vi "PC_Record.vi"() -> ()   [LabVIEW 2018]
uses:
  <vilib>/Utility/inputDevices.llb/joystickAcquire.vi
  <vilib>/Utility/file.llb/Write Delimited Spreadsheet (DBL).vi
  <vilib>/Utility/inputDevices.llb/closeJoystick.vi
  <resource>/objmgr/ni.dex.rc
panel:
  out "output cluster":T1
  out "output array":dbl[](array[numeric])
  out "direction info":T2
  in  "file path (dialog if empty)":path=path "C:/Users/Silvis/Desktop/file01"
  in  "myRIO IP address":string(combo)
  out "timed out?":bool
  in  "Stop Button":bool
  out "RT reader URL":string="///RT-reader"
  out "RT connected?":bool
  out "error out 2":errorcluster
  # "PC host writer"
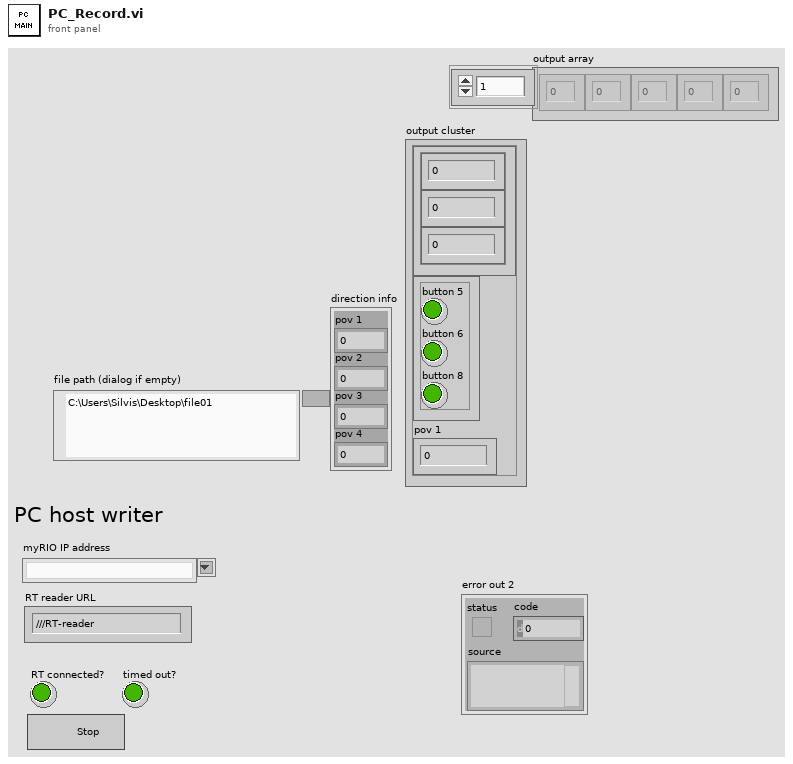
[diagram p1: front panel]
types:
  T1 = cluster{"Cluster":cluster{"Numeric Control":dbl, "Numeric Control":dbl, "Numeric Control":dbl}, "Cluster":cluster{"button 5":bool, "button 6":bool, "button 8":bool}, "pov 1":i32}
  T2 = cluster{"pov 1":i32, "pov 2":i32, "pov 3":i32, "pov 4":i32}
  T3 = cluster{"X axis":i32, "Y axis":i32, "Z axis":i32, "X axis rotation":i32, "Y axis rotation":i32, "Z axis rotation":i32, "U axis":i32, "V axis":i32}
  T4 = cluster{"button 1":bool, "button 2":bool, "button 3":bool, "button 4":bool, "button 5":bool, "button 6":bool, "button 7":bool, "button 8":bool, "button 9":bool, "button 10":bool, "button 11":bool, "button 12":bool, "button 13":bool, "button 14":bool, "button 15":bool, "button 16":bool, "button 17":bool, "button 18":bool, "button 19":bool, "button 20":bool, "button 21":bool, "button 22":bool, "button 23":bool, "button 24":bool, "button 25":bool, "button 26":bool, "button 27":bool, "button 28":bool, "button 29":bool, "button 30":bool, "button 31":bool, "button 32":bool}
  T5 = cluster{"button 5":bool, "button 6":bool, "button 8":bool}
  T6 = cluster{cluster{dbl, dbl, dbl}, cluster{"button 5":bool, "button 6":bool, "button 8":bool}, "pov 1":i32}
  T7 = cluster{"Cluster":cluster{"Numeric Control":dbl, "Numeric Control":dbl, "Numeric Control":dbl}, "Cluster":cluster{"button 5":bool, "button 6":bool, "button 8":bool}, "pov 1":i32}[]
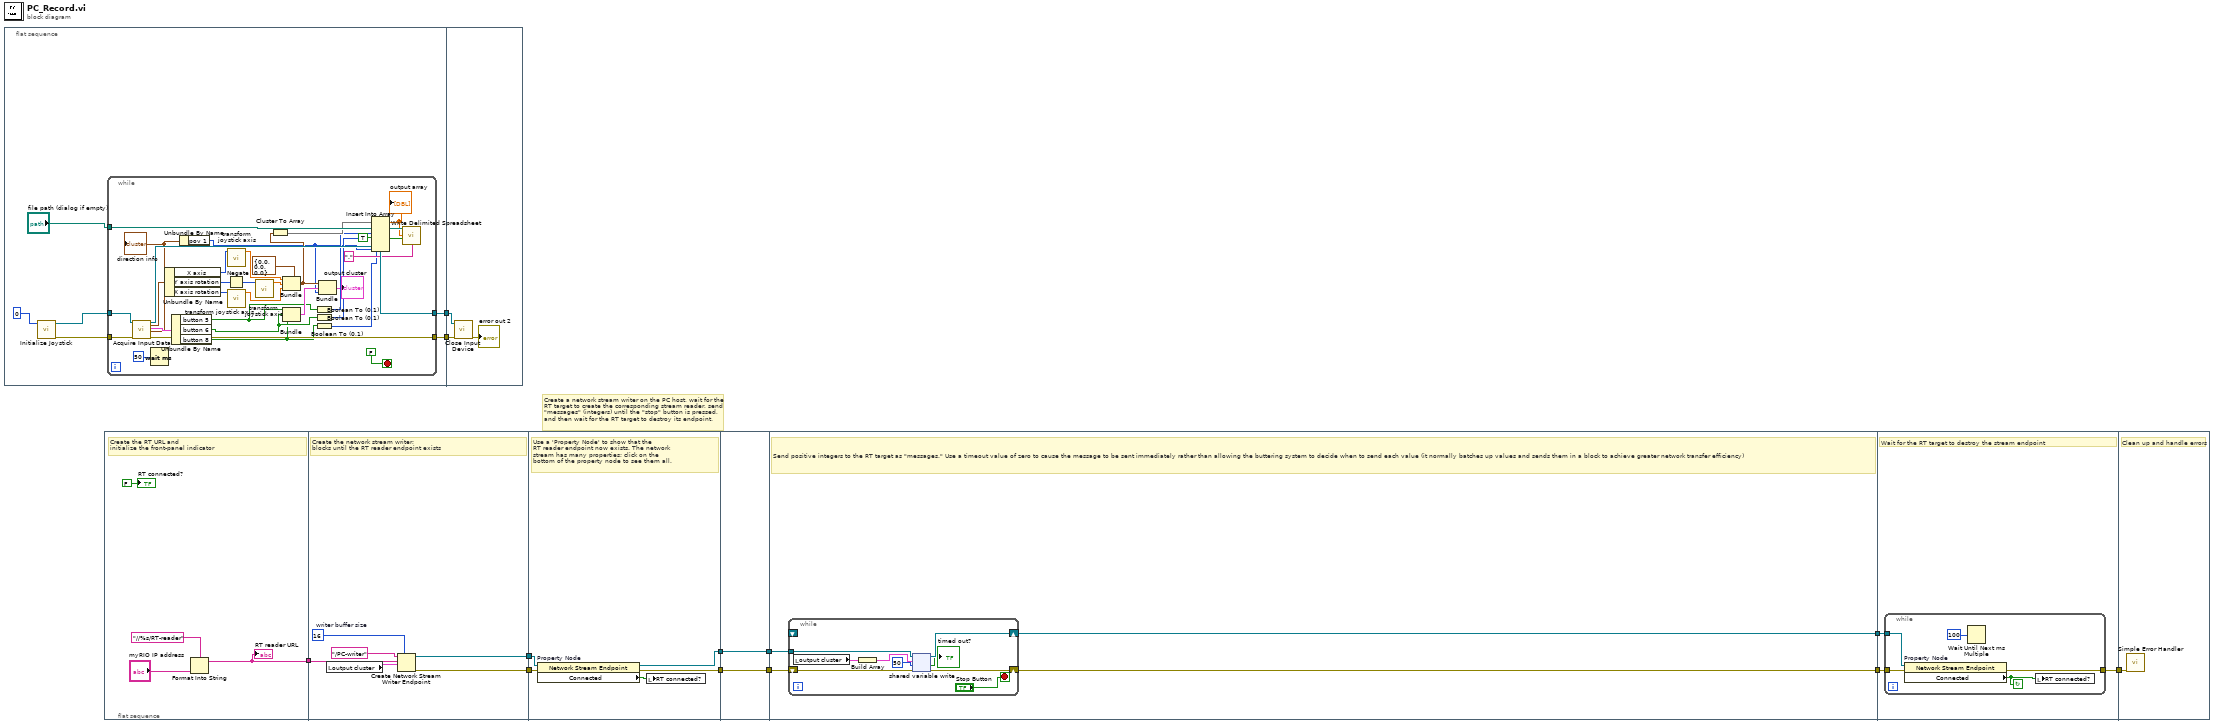
[diagram p0: block diagram]
diagram:
  # "Create a network stream writer on the PC host, wait for the\nRT target to create the corresponding stream reader, send\n\"messages\" (integers) until the \"stop\" button is pressed,\nand then wait for the RT target to destroy its endpoint."
  n1 = flat-sequence {
    tunnel: [w16] -> w2
    tunnel: [w15] -> w1
    tunnel: w2 -> [w53]
    tunnel: w1 -> [w52]
    frame #0 {
      n2 = call <vilib>:"Initialize Joystick.vi"("device index"=0) -> ("error out"=w17:errorcluster, "device ID"=w18:refnum<k1>)  [unwired: 9 in]
      n3 = while {
        tunnel: w18 -> [w50]
        tunnel: w17 -> [w49]
        tunnel: [w48] -> w16
        tunnel: [w29] -> w15
        tunnel: "file path (dialog if empty)" -> [w46]
        stop <- FALSE stop-if-true
        n4 = call-poly <vilib>:"Acquire Input Data.vi"("device ID"=w50, "error in (no error)"=w49) -> ("device ID"=w48:refnum<k1>, "axis info"=w40:T3, "button info"=w39:T4, "direction info"=w22:T2, "error out"=w29:errorcluster)  [unwired: 13 in]
        "direction info" <- w22
        n5 = Wait (ms)(milliseconds to wait=u32 50) -> ()  [unwired: 1 out]
        n6 = Unbundle By Name(w40) -> ("X axis"=w43:i32, "Y axis rotation"=w44:i32, "X axis rotation"=w41:i32)
        n7 = Unbundle By Name(w39) -> ("button 5"=w30:bool, "button 6"=w28:bool, "button 8"=w27:bool)
        n8 = Unbundle By Name(w22) -> ("pov 1"=w20:i32)
        n9 = Negate(x=w44) -> (-x=w42:i32)
        n10 = call <vilib>:"transform joystick axis.vi"("Axis Input"=w43) -> ("Output (-1..1)"=w37:dbl)  [unwired: 10 in]
        n11 = call <vilib>:"transform joystick axis.vi"("Axis Input"=w41) -> ("Output (-1..1)"=w35:dbl)  [unwired: 10 in]
        n12 = call <vilib>:"transform joystick axis.vi"("Axis Input"=w42) -> ("Output (-1..1)"=w36:dbl)  [unwired: 10 in]
        n13 = Bundle(cluster=cluster{dbl, dbl, dbl} {0.0, 0.0, 0.0}, w37, w36, w35) -> (w34:cluster{dbl, dbl, dbl})
        n14 = Cluster To Array(cluster=w34) -> (array=w26:dbl[])
        n15 = Bundle("button 5"=w30, "button 6"=w28, "button 8"=w27) -> (w31:T5)  [unwired: 1 in]
        n16 = Boolean To (0,1)(Boolean=w30) -> (0, 1=w25:i16)
        n17 = Boolean To (0,1)(Boolean=w28) -> (0, 1=w24:i16)
        n18 = Boolean To (0,1)(Boolean=w27) -> (0, 1=w23:i16)
        n19 = Bundle(w34, w31, "pov 1"=w20) -> (→"output cluster":T6)  [unwired: 1 in]
        n20 = Insert Into Array(array=w26, new element #1=w25, new element #2=w24, new element #3=w23, new element #4=w20) -> (w21:dbl[])  [unwired: 1 in]
        "output array" <- w21
        n21 = call-poly <vilib>:"Write Delimited Spreadsheet.vi"("file path (dialog if empty)"=w46, "1D data"=w21, "append to file? (new file:F)"=TRUE, "delimiter (\\t)"="." ("delimiter (\\t)")) -> ()  [unwired: 10 in, 2 out]
      }
    }
    frame #1 {
      n22 = call-poly <vilib>:"Close Input Device.vi"("error in (no error)"=w52, "device ID"=w53) -> ("error out"=→"error out 2":errorcluster)  [unwired: 8 in]
    }
  }
  n23 = flat-sequence {
    tunnel: [w56] -> w12
    tunnel: w12 -> [w61]
    tunnel: [w60] -> w11
    tunnel: [w59] -> w10
    tunnel: w11 -> [w68]
    tunnel: w10 -> [w67]
    tunnel: [w66] -> w6
    tunnel: [w65] -> w4
    tunnel: w6 -> [w70]
    tunnel: [w70] -> w5
    tunnel: w4 -> [w69]
    tunnel: [w69] -> w3
    tunnel: w5 -> [w74]
    tunnel: w3 -> [w73]
    tunnel: [w72] -> w9
    tunnel: [w71] -> w8
    tunnel: w9 -> [w86]
    tunnel: w8 -> [w85]
    tunnel: [w84] -> w7
    tunnel: w7 -> [w92]
    frame #0 {
      # "Create the RT URL and\ninitialize the front-panel indicator"
      n24 = Format Into String "Format Into String"(format string="//%s/RT-reader", "myRIO IP address") -> (resulting string=w56:string)  [unwired: 2 in, 1 out]
      "RT reader URL" <- w56
      "RT connected?" <- FALSE ("RT connected?")
    }
    frame #1 {
      w63 = 16  # writer buffer size
      # "Create the network stream writer;\nblocks until the RT reader endpoint exists"
      n25 = local read "output cluster"() -> (w58:T1)
      n26 = Create Network Stream Writer Endpoint(7:w63, 9:w58, 10:w61, 11:"/PC-writer" ("writer name")) -> (0:w59:errorcluster, 3:w60:refnum<k21>)  [unwired: 3 in]
    }
    frame #2 {
      # "Use a 'Property Node' to show that the\nRT reader endpoint now exists. The network\nstream has many properties; click on the\nbottom of the property node to see them all."
      n27 = property on="Property Node" class="Network Stream Endpoint"(reference=w68, error in=w67) -> (reference out=w66:refnum<k21>, error out=w65:errorcluster, "Connected"=w64:bool)
      n28 = local write "RT connected?"(w64) -> ()
    }
    frame #3 {
    }
    frame #4 {
      # "Send positive integers to the RT target as \"messages.\" Use a timeout value of zero to cause the message to be sent immediately rather than allowing the buttering system to decide when to send each value (it normally batches up values and sends them in a block to achieve greater network transfer efficiency)"
      n29 = while {
        shift-right: [w79] -> w71
        shift-left: w73 -> [w80]
        tunnel: w74 -> [w82]
        shift-right: [w78] -> w72
        shift-left: _ -> [_]
        stop <- "Stop Button" stop-if-true
        n30 = local read "output cluster"() -> (w76:T1)
        n31 = Build Array(w76) -> (w75:T7)
        n32 = shared-variable-write(w82, w80, w75, 50 ("timeout ms (-1)")) -> (w78:refnum<k21>, w79:errorcluster, →"timed out?":bool)
      }
    }
    frame #5 {
      # "Wait for the RT target to destroy the stream endpoint"
      n33 = while {
        tunnel: w86 -> [w91]
        tunnel: w85 -> [w90]
        tunnel: [w89] -> w84
        stop <- w87 continue-if-true
        # "wait for RT to destroy the endpoint"
        n34 = property on="Property Node" class="Network Stream Endpoint"(reference=w91, error in=w90) -> (error out=w89:errorcluster, "Connected"=w87:bool)  [unwired: 1 out]
        n35 = Wait Until Next ms Multiple(millisecond multiple=u32 100) -> ()  [unwired: 1 out]
        n36 = local write "RT connected?"(w87) -> ()
      }
    }
    frame #6 {
      # "Clean up and handle errors"
      n37 = call <vilib>:"Simple Error Handler.vi"("error in (no error)"=w92) -> ()  [unwired: 4 in, 5 out]
    }
  }
